vi "sample obtain and delete bucket.vi"() -> ()   [LabVIEW 2015]
uses:
  Core/HTTP Request/Region.ctl
  Bucket/Versioning Status.ctl
  Bucket/MFA Delete.ctl
  Auth Device Data.ctl
  Core/HTTP Request/AWS Credentials.ctl
  Bucket/Bucket.lvclass
  Core/HTTP Request/HTTP Request.lvclass
  NI_AWS_S3.lvlib
panel:
  in  "Auth device data":T1
  out "MFA Delete":T2
  out "Status":T3
  out "Location":T4
  out "error out":errorcluster
  in  "Bucket name":string="bpreis-test-95"
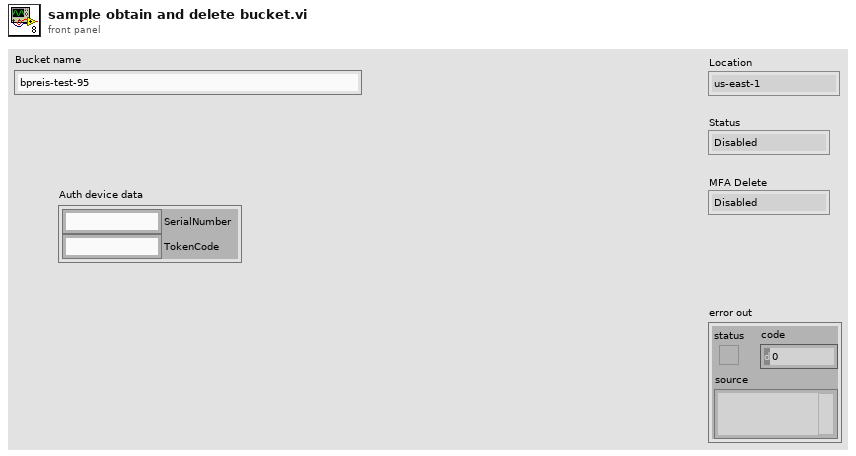
[diagram p1: front panel]
types:
  T1 = typedef "NI_AWS_S3.lvlib/Auth Device Data.ctl" = cluster{"SerialNumber":string, "TokenCode":string}
  T2 = typedef "NI_AWS_S3.lvlib/Bucket.lvclass/MFA Delete.ctl" = enum16{"Disabled", "Enabled"}
  T3 = typedef "NI_AWS_S3.lvlib/Bucket.lvclass/Versioning Status.ctl" = enum16{"Disabled", "Suspended", "Enabled"}
  T4 = typedef "NI_AWS_Core.lvlib/HTTP Request.lvclass/Region.ctl" = enum16{"us-east-1", "us-east-2", "us-west-1", "us-west-2", "ap-northeast-1", "ap-northeast-2", "ap-southeast-1", "ap-southeast-2", "ca-central-1", "eu-central-1", "eu-west-1", "eu-west-2", "sa-east-1"}
  T5 = typedef "NI_AWS_Core.lvlib/HTTP Request.lvclass/AWS Credentials.ctl" = cluster{"Access Key":string, "Secret Key":string}
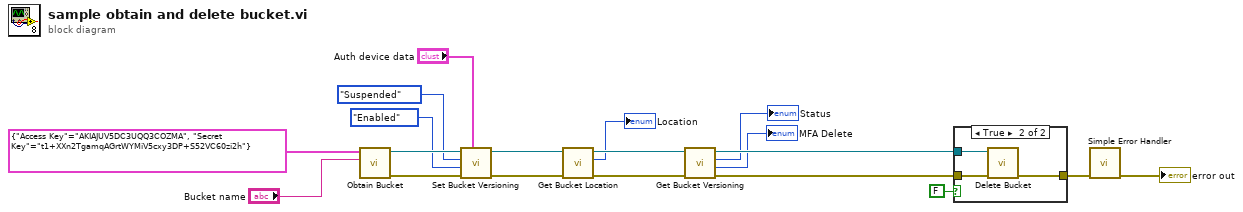
[diagram p0: block diagram]
diagram:
  n1 = call "Obtain Bucket.vi"("Bucket name"="Bucket name", "AWS Credentials"=T5 {"Access Key"="AKIAJUV5DC3UQQ3COZMA", "Secret Key"="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"}) -> ("error out"=w19:errorcluster, "Bucket"=w5:refnum<class "Bucket.lvclass">)  [unwired: 8 in]
  n2 = call "Set Bucket Versioning.vi"("Auth device data"="Auth device data", "error in (no error)"=w19, "MFA Delete"=MFA_Delete."Enabled", "Status"=Versioning_Status."Suspended", "Bucket in"=w5) -> ("error out"=w6:errorcluster, "Bucket out"=w4:refnum<class "Bucket.lvclass">)  [unwired: 5 in]
  n3 = call "Get Bucket Location.vi"("error in (no error)"=w6, "Bucket in"=w4) -> ("error out"=w14:errorcluster, "Location"=→"Location":T4, "Bucket out"=w12:refnum<class "Bucket.lvclass">)  [unwired: 7 in]
  n4 = call "Get Bucket Versioning.vi"("error in (no error)"=w14, "Bucket in"=w12) -> ("error out"=w13:errorcluster, "MFA Delete"=→"MFA Delete":T2, "Status"=→"Status":T3, "Bucket out"=w11:refnum<class "Bucket.lvclass">)  [unwired: 6 in]
  n5 = case shown="True" FALSE {
    tunnel: [w20 w23] -> w18
    tunnel: w13 -> [w20 w22]
    tunnel: w11 -> [_ w21]
    frame False {
    }
    frame True {
      n6 = call "Delete Bucket.vi"("error in (no error)"=w22, "Bucket in"=w21) -> ("error out"=w23:errorcluster)  [unwired: 9 in]
    }
  }
  n7 = call <vilib>:"Simple Error Handler.vi"("error in (no error)"=w18) -> ("error out"=→"error out":errorcluster)  [unwired: 4 in, 4 out]
